vi "Explode.vi"(8 "error in (no error)":errorcluster, 11 "SnailNum in":refnum<class "SnailNum.lvclass">) -> (0 "error out":errorcluster, 2 "Explode Result":T1, 3 "SnailNum out":refnum<class "SnailNum.lvclass">)   [LabVIEW 2020, in "SnailNum.lvclass"]
uses:
  SnailNum.lvclass
  Explode Result.ctl
  SnailNum.lvclass/SnailNum.ctl
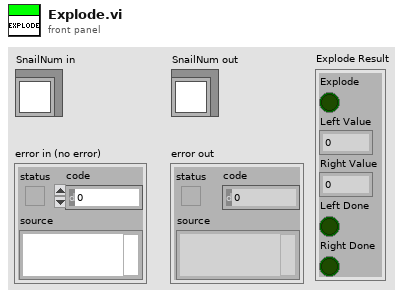
[diagram p1: front panel]
types:
  T1 = typedef "SnailNum.lvclass/Explode Result.ctl" = cluster{"Explode":bool, "Left Value":i64, "Right Value":i64, "Left Done":bool, "Right Done":bool}
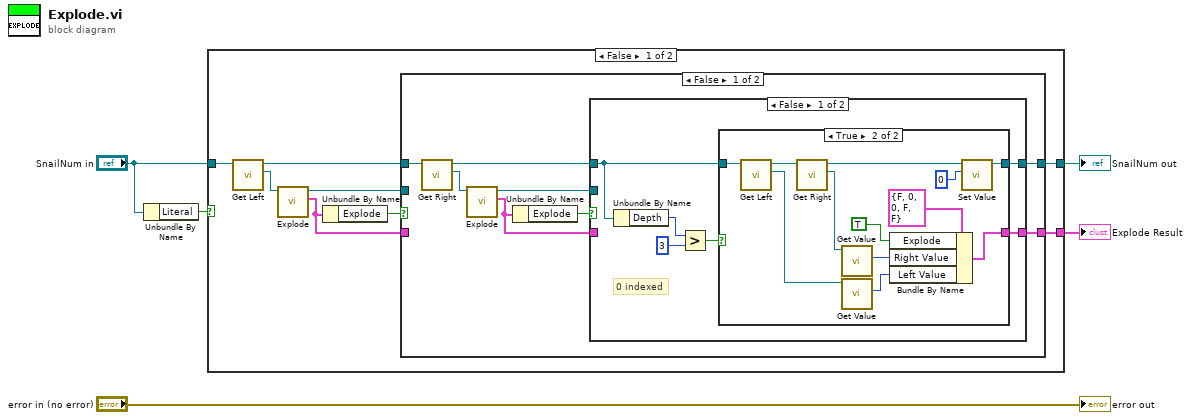
[diagram p0: block diagram]
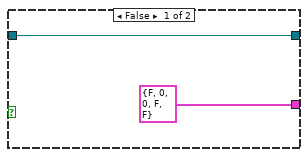
[diagram p2: hidden frame]
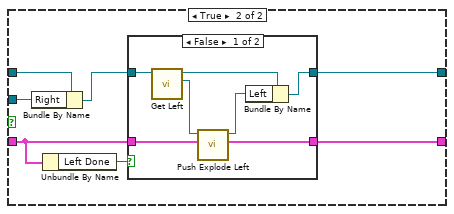
[diagram p3: hidden frame]
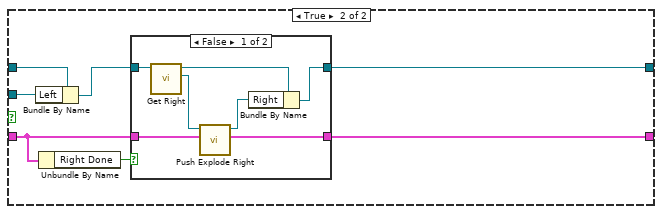
[diagram p5: hidden frame]
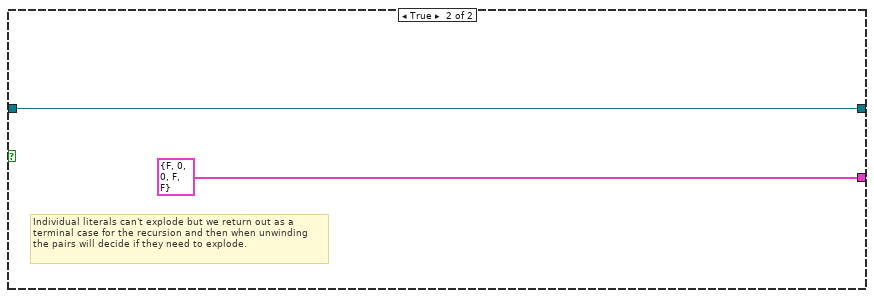
[diagram p7: hidden frame]
diagram:
  n1 = Unbundle By Name("SnailNum in") -> ("Literal"=w4:bool)
  n2 = case shown="False" w4 {
    tunnel: "SnailNum in" -> [w13 w75]
    tunnel: [w6 w75] -> w2
    tunnel: [w7 T1 {"Explode"=FALSE, "Left Value"=0, "Right Value"=0, "Left Done"=FALSE, "Right Done"=FALSE} ("Explode Result")] -> w1
    frame False {
      n3 = call "Get Left.vi"("SnailNum in"=w13) -> ("Left"=w12:refnum<class "SnailNum.lvclass">, "SnailNum out"=w10:refnum<class "SnailNum.lvclass">)  [unwired: 8 in, 1 out]
      n4 = call "Explode.vi"("SnailNum in"=w12) -> ("Explode Result"=w8:T1, "SnailNum out"=w9:refnum<class "SnailNum.lvclass">)  [unwired: 8 in, 1 out]
      n5 = Unbundle By Name(w8) -> ("Explode"=w11:bool)
      n6 = case shown="False" w11 {
        tunnel: w10 -> [w21 w63]
        tunnel: w9 -> [_ w58]
        tunnel: w8 -> [_ w62]
        tunnel: [w14 w61] -> w7
        tunnel: [w15 w60] -> w6
        frame False {
          n7 = call "Get Right.vi"("SnailNum in"=w21) -> ("Right"=w20:refnum<class "SnailNum.lvclass">, "SnailNum out"=w18:refnum<class "SnailNum.lvclass">)  [unwired: 8 in, 1 out]
          n8 = call "Explode.vi"("SnailNum in"=w20) -> ("Explode Result"=w16:T1, "SnailNum out"=w19:refnum<class "SnailNum.lvclass">)  [unwired: 8 in, 1 out]
          n9 = Unbundle By Name(w16) -> ("Explode"=w17:bool)
          n10 = case shown="False" w17 {
            tunnel: w19 -> [_ w48]
            tunnel: w18 -> [w25 w46]
            tunnel: w16 -> [_ w43]
            tunnel: [w23 w45] -> w15
            tunnel: [w22 w42] -> w14
            frame False {
              # "0 indexed"
              n11 = Unbundle By Name(w25) -> ("Depth"=w27:i32)
              n12 = Greater?(x=w27, y=3) -> (0:w24:bool)
              n13 = case shown="True" w24 {
                tunnel: w25 -> [w28 w41]
                tunnel: [w28 w32] -> w23
                tunnel: [T1 {"Explode"=FALSE, "Left Value"=0, "Right Value"=0, "Left Done"=FALSE, "Right Done"=FALSE} ("Explode Result") w34] -> w22
                frame False {
                }
                frame True {
                  n14 = call "Get Left.vi"("SnailNum in"=w41) -> ("Left"=w39:refnum<class "SnailNum.lvclass">, "SnailNum out"=w40:refnum<class "SnailNum.lvclass">)  [unwired: 8 in, 1 out]
                  n15 = call "Get Right.vi"("SnailNum in"=w40) -> ("Right"=w38:refnum<class "SnailNum.lvclass">, "SnailNum out"=w33:refnum<class "SnailNum.lvclass">)  [unwired: 8 in, 1 out]
                  n16 = call "Get Value.vi"("SnailNum in"=w38) -> ("Value"=w36:i64)  [unwired: 8 in, 2 out]
                  n17 = call "Get Value.vi"("SnailNum in"=w39) -> ("Value"=w35:i64)  [unwired: 8 in, 2 out]
                  n18 = Bundle By Name(cluster=T1 {"Explode"=FALSE, "Left Value"=0, "Right Value"=0, "Left Done"=FALSE, "Right Done"=FALSE} ("Explode Result"), "Explode"=TRUE, "Right Value"=w36, "Left Value"=w35) -> (w34:T1)
                  n19 = call "Set Value.vi"("Value"=i64 0, "SnailNum in"=w33) -> ("SnailNum out"=w32:refnum<class "SnailNum.lvclass">)  [unwired: 8 in, 1 out]
                }
              }
            }
            frame True {
              n20 = Bundle By Name(cluster=w46, "Right"=w48) -> (w44:refnum<class "SnailNum.lvclass">)
              n21 = Unbundle By Name(w43) -> ("Left Done"=w47:bool)
              n22 = case shown="False" w47 {
                tunnel: w44 -> [w55 w57]
                tunnel: [w50 w57] -> w45
                tunnel: w43 -> [w53 w56]
                tunnel: [w51 w56] -> w42
                frame False {
                  n23 = call "Get Left.vi"("SnailNum in"=w55) -> ("Left"=w52:refnum<class "SnailNum.lvclass">, "SnailNum out"=w54:refnum<class "SnailNum.lvclass">)  [unwired: 8 in, 1 out]
                  n24 = call "Push Explode Left.vi"("Explode Result In"=w53, "SnailNum in"=w52) -> ("Explode Result"=w51:T1, "SnailNum out"=w49:refnum<class "SnailNum.lvclass">)  [unwired: 7 in, 1 out]
                  n25 = Bundle By Name(cluster=w54, "Left"=w49) -> (w50:refnum<class "SnailNum.lvclass">)
                }
                frame True {
                }
              }
            }
          }
        }
        frame True {
          n26 = Bundle By Name(cluster=w63, "Left"=w58) -> (w59:refnum<class "SnailNum.lvclass">)
          n27 = Unbundle By Name(w62) -> ("Right Done"=w64:bool)
          n28 = case shown="False" w64 {
            tunnel: w59 -> [w71 w73]
            tunnel: w62 -> [w68 w72]
            tunnel: [w67 w72] -> w61
            tunnel: [w69 w73] -> w60
            frame False {
              n29 = call "Get Right.vi"("SnailNum in"=w71) -> ("Right"=w66:refnum<class "SnailNum.lvclass">, "SnailNum out"=w70:refnum<class "SnailNum.lvclass">)  [unwired: 8 in, 1 out]
              n30 = call "Push Explode Right.vi"("Explode Result In"=w68, "SnailNum in"=w66) -> ("Explode Result"=w67:T1, "SnailNum out"=w65:refnum<class "SnailNum.lvclass">)  [unwired: 7 in, 1 out]
              n31 = Bundle By Name(cluster=w70, "Right"=w65) -> (w69:refnum<class "SnailNum.lvclass">)
            }
            frame True {
            }
          }
        }
      }
    }
    frame True {
      # "Individual literals can't explode but we return out as a terminal case for the recursion and then when unwinding the pairs will decide if they need to explode."
    }
  }
  "SnailNum out" <- w2
  "Explode Result" <- w1
  "error out" <- "error in (no error)"
